vi "SET_INPUT_GAINS_n.vi"(2 "execute":bool, 5 "G1":u8(slide) scale=0.0..3.0, 9 "G2":u8(slide) scale=0.0..3.0, 11 "error in (no error)":errorcluster) -> (4 "function return":string, 15 "error out":errorcluster)   [LabVIEW 2017, in "ZBOX_IS.lvlib"]
uses:
  ZBOX_IS.lvlib
panel:
  # "10"
  # "5"
  # "2"
  # "1"
  # "10"
  # "5"
  # "2"
  # "1"
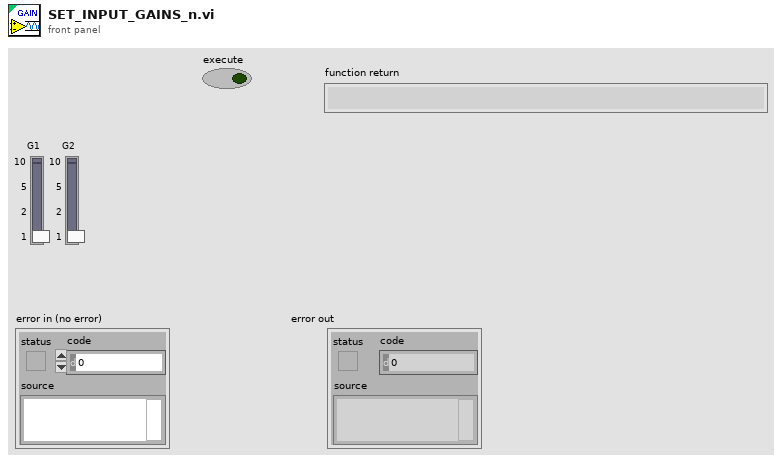
[diagram p1: front panel]
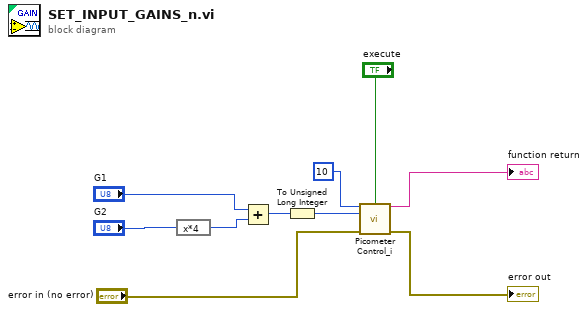
[diagram p0: block diagram]
diagram:
  n1 = expression code="x*4"("G2") -> (w6:u8)
  n2 = Add(x="G1", y=w6) -> (x+y=w5:u8)
  n3 = To Unsigned Long Integer(number=w5) -> (unsigned 32bit integer=w4:u32)
  n4 = call "Picometer Control_i.vi"("Cmd"=u8 10, "execute"="execute", "ulValue"=w4, "error in (no error)"="error in (no error)") -> ("function return"=→"function return":string, "error out"=→"error out":errorcluster)  [unwired: 7 in, 3 out]
